vi "gentec-M-Link.Read.vi"(0 "VISA resource (In)":refnum<visa-resource-name>, 5 "error in (no error)":errorcluster) -> (14 "VISA resource (Out)":refnum<visa-resource-name>, 16 "Data Read":string, 17 "Bytes Read":u32, 18 "Read Timeout":bool, 19 "error out":errorcluster)   [LabVIEW 2014, in "gentec-M-Link - Driver.lvlib"]
doc: "This VI calls a VISA Read."
uses:
  gentec-M-Link - Driver.lvlib
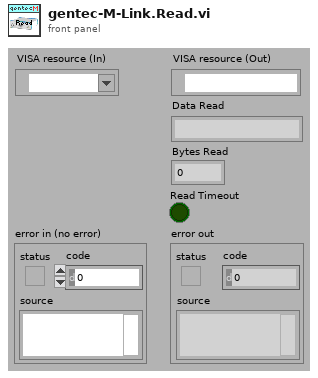
[diagram p1: front panel]
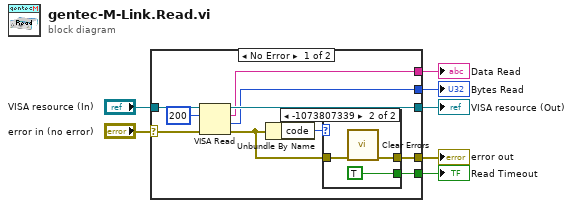
[diagram p0: block diagram]
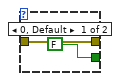
[diagram p2: hidden frame]
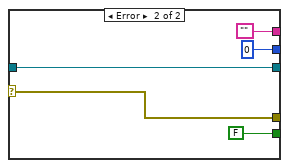
[diagram p3: hidden frame]
diagram:
  n1 = case shown="No Error" "error in (no error)" {
    selector: "error in (no error)" -> [w17 w27]
    tunnel: [w9 w27] -> w6
    tunnel: "VISA resource (In)" -> [w16 w26]
    tunnel: [w15 w26] -> w4
    tunnel: [w12 ""] -> w3
    tunnel: [w8 FALSE] -> w2
    tunnel: [w13 u32 0 ("return count")] -> w1
    frame No Error {
      n2 = VISA Read(VISA resource name=w16, byte count=u32 200, error in (no error)=w17) -> (VISA resource name out=w15:refnum<visa-resource-name>, read buffer=w12:string, return count=w13:u32, error out=w10:errorcluster)
      n3 = Unbundle By Name(w10) -> ("code"=w11:i32)
      n4 = case shown="-1073807339" w11 {
        tunnel: w10 -> [w19 w20]
        tunnel: [w19 w21] -> w9
        tunnel: [FALSE TRUE] -> w8
        frame 0, Default {
        }
        frame -1073807339 {
          n5 = call <vilib>:"Clear Errors.vi"("error in (no error)"=w20) -> ("error out"=w21:errorcluster)  [unwired: 5 in, 1 out]
        }
      }
    }
    frame Error {
    }
  }
  "error out" <- w6
  "VISA resource (Out)" <- w4
  "Data Read" <- w3
  "Read Timeout" <- w2
  "Bytes Read" <- w1
